vi "AnalyzeCalibrations.vi"() -> ()   [LabVIEW 2019, in "Analysis.lvlib"]
uses:
  Analysis.lvlib
  <vilib>/ptbypt/NI_PtbyPt.lvlib
  <vilib>/Analysis/NI_AALBase.lvlib
panel:
  out "Error Out":errorcluster
  in  "Error In":errorcluster
  in  "Analysis":T1(tab)
  in  "Exit Button":bool
  in  "Offset Histo Plot Button":bool
  out "Sample Size":dbl format="%#_4g"
  out "Max":dbl format="%.3g"
  out "Min":dbl format="%.3g"
  out "Mean":dbl format="%.3g"
  out "Std Deviation":dbl format="%.3g"
  out "Histogram Graph":T2(graph)
  in  "XML File Path":path=path "C:/users/CIL/Documents/LabVIEW Data/Aquatrak Data"
  in  "Exit Button 2":bool
  out "Offset Values vs. Time":cluster{timestamp[], dbl[]}[](graph)
  in  "Time vs Offset":bool
  in  "Exit Button 3":bool
  out "Sample Size":dbl format="%_2g"
  out "Max Temp":dbl format="%.3g"
  out "MinTemp":dbl format="%.3g"
  out "Mean Temp":dbl format="%.3g"
  in  "Offset vs. Temp":bool
  out "Offset vs. Temperature":cluster{dbl[], dbl[]}(graph)
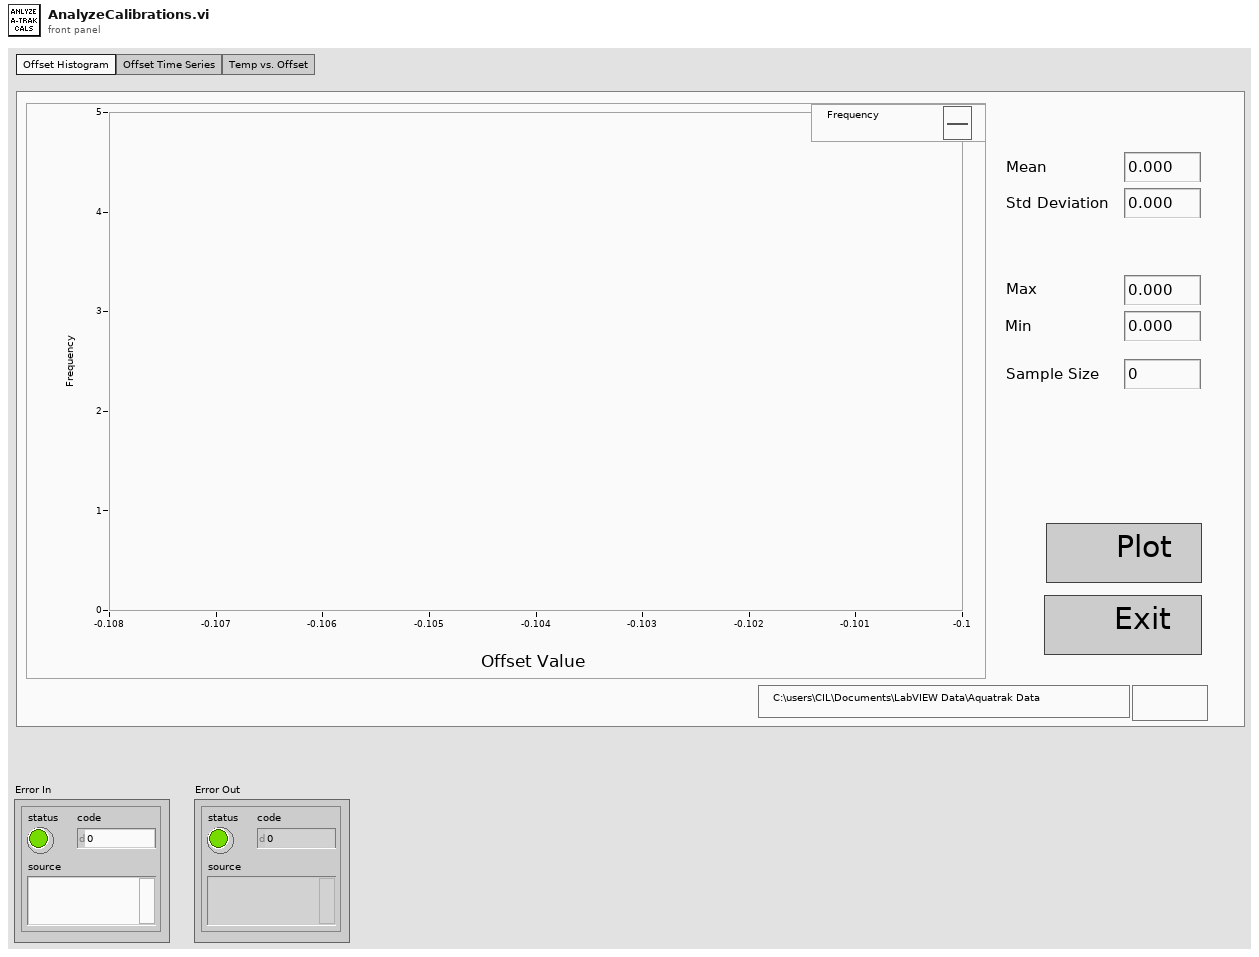
[diagram p1: front panel]
types:
  T1 = enum32{"Offset Histogram", "Offset Time Series", "Temp vs. Offset"}
  T2 = cluster{"X Values":dbl[], "Histogram: h(x)":i32[]}
  T3 = cluster{timestamp[], string[], string[], string[], string[], dbl[], dbl[], dbl[], "SSC Out (meters)":dbl[][], dbl[], dbl[], dbl[]}
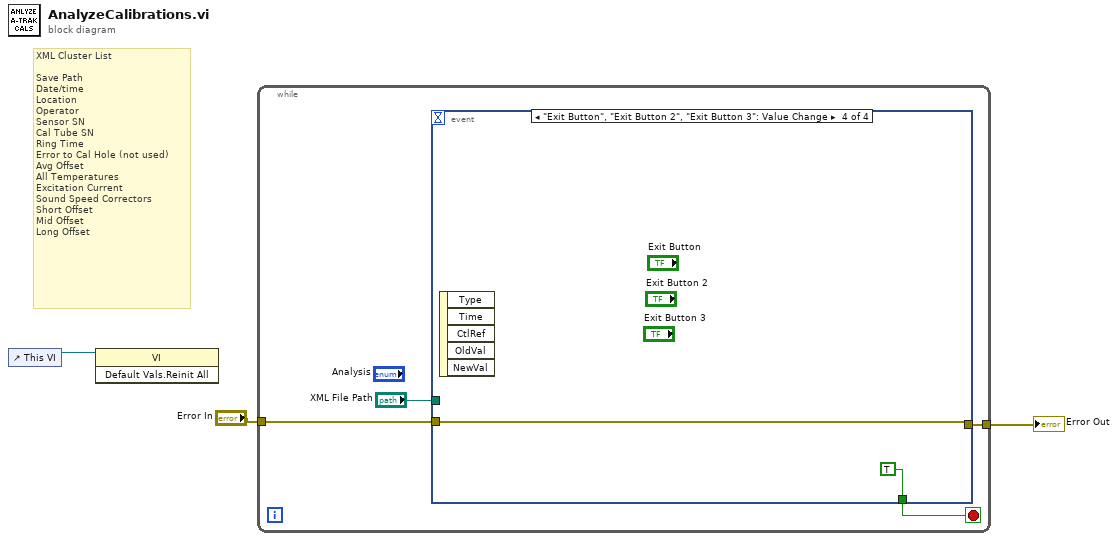
[diagram p0: block diagram]
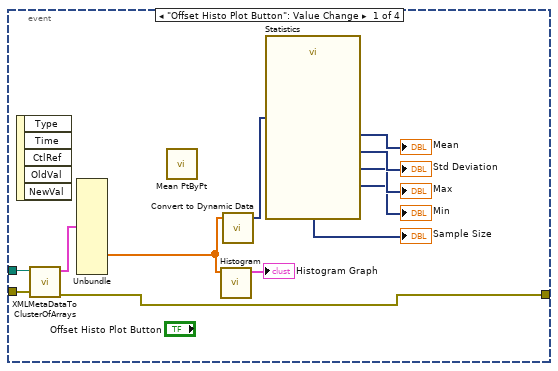
[diagram p2: hidden frame]
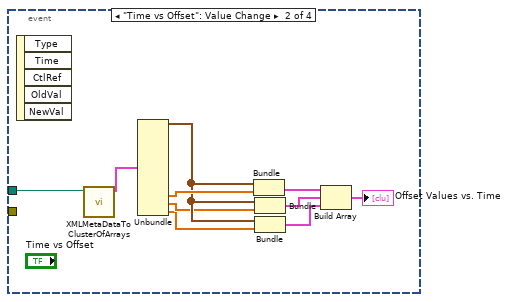
[diagram p3: hidden frame]
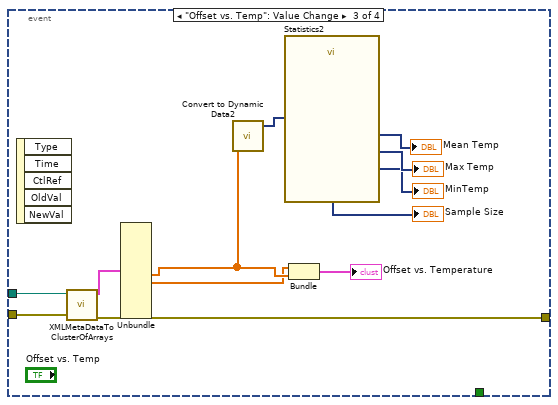
[diagram p4: hidden frame]
diagram:
  # "XML Cluster List\n\nSave Path\nDate/time\nLocation\nOperator\nSensor SN\nCal Tube SN\nRing Time\nError to Cal Hole (not used)\nAvg Offset\nAll Temperatures\nExcitation Current\nSound Speed Correctors\nShort Offset\nMid Offset\nLong Offset"
  n1 = control-ref of="This VI"() -> (w1:refnum<vi>)
  n2 = invoke class="VI" method="Default Vals.Reinit All"(reference=w1) -> ()  [unwired: 2 in, 3 out]
  n3 = while {
    tunnel: "Error In" -> [w5]
    tunnel: [w4] -> w2
    stop <- w6 stop-if-true
    n4 = event shown="[3] \"Exit Button\", \"Exit Button 2\", \"Exit Button 3\": Value Change" {
      selector: _ -> [_ _ _ _]
      dyn-events: _ -> [_ _ _ _]
      timeout: _ -> [_ _ _ _]
      tunnel: "XML File Path" -> [w19 w28 w40 _]
      tunnel: [_ _ _ TRUE] -> w6
      tunnel: w5 -> [w11 _ w39 w42]
      tunnel: [w9 _ w33 w42] -> w4
      event "Offset Histo Plot Button": Value Change {
        n5 = event-data() -> ()  [unwired: 1 in, 5 out]
        n6 = call "XMLMetaDataToClusterOfArrays.vi"("error in"=w11, "XML File Path"=w19) -> ("error out"=w9:errorcluster, "Results Cluster"=w18:T3)  [unwired: 7 in, 1 out]
        n7 = Unbundle(w18) -> (w10:dbl[])  [unwired: 11 out]
        n8 = call <vilib>:"Mean PtByPt.vi"() -> ()  [unwired: 4 in, 2 out]
        n9 = call <vilib>:"Histogram.vi"("X"=w10) -> ("Histogram Graph"=→"Histogram Graph":T2)  [unwired: 7 in, 3 out]
        n10 = call "Convert to Dynamic Data"("Array"=w10) -> ("Dynamic Data Type"=w17:dynamicdata)  [unwired: 3 in]
        n11 = call "Statistics"("Signals"=w17) -> ("Total Samples"=→"Sample Size":dynamicdata, "Standard Dev"=→"Std Deviation":dynamicdata, "Arithmetic Mean"=→"Mean":dynamicdata, "Minimum"=→"Min":dynamicdata, "Maximum"=→"Max":dynamicdata)  [unwired: 21 in, 1 out]
      }
      event "Time vs Offset": Value Change {
        n12 = event-data() -> ()  [unwired: 1 in, 5 out]
        n13 = call "XMLMetaDataToClusterOfArrays.vi"("XML File Path"=w28) -> ("Results Cluster"=w29:T3)  [unwired: 8 in, 2 out]
        n14 = Unbundle(w29) -> (w26:timestamp[], w27:dbl[], w25:dbl[], w24:dbl[])  [unwired: 8 out]
        n15 = Bundle(w26, w27) -> (w23:cluster{timestamp[], dbl[]})  [unwired: 1 in]
        n16 = Bundle(w26, w25) -> (w22:cluster{timestamp[], dbl[]})  [unwired: 1 in]
        n17 = Bundle(w26, w24) -> (w21:cluster{timestamp[], dbl[]})  [unwired: 1 in]
        n18 = Build Array(w23, w22, w21) -> (→"Offset Values vs. Time":cluster{timestamp[], dbl[]}[])
      }
      event "Offset vs. Temp": Value Change {
        n19 = event-data() -> ()  [unwired: 1 in, 5 out]
        n20 = call "XMLMetaDataToClusterOfArrays.vi"("error in"=w39, "XML File Path"=w40) -> ("error out"=w33:errorcluster, "Results Cluster"=w41:T3)  [unwired: 7 in, 1 out]
        n21 = Unbundle(w41) -> (w31:dbl[], w30:dbl[])  [unwired: 10 out]
        n22 = call "Convert to Dynamic Data2"("Array"=w31) -> ("Dynamic Data Type"=w38:dynamicdata)  [unwired: 3 in]
        n23 = call "Statistics2"("Signals"=w38) -> ("Total Samples"=→"Sample Size":dynamicdata, "Arithmetic Mean"=→"Mean Temp":dynamicdata, "Minimum"=→"MinTemp":dynamicdata, "Maximum"=→"Max Temp":dynamicdata)  [unwired: 21 in, 2 out]
        n24 = Bundle(w30, w31) -> (→"Offset vs. Temperature":cluster{dbl[], dbl[]})  [unwired: 1 in]
      }
      event "Exit Button", "Exit Button 2", "Exit Button 3": Value Change {
        n25 = event-data() -> ()  [unwired: 1 in, 5 out]
      }
    }
  }
  "Error Out" <- w2
